vi "Sequencer Main - Copy.vi"() -> ()   [LabVIEW 2018] (continued)
                            }
                          }
                        }
                        frame 47 {
                          # "FALSE/Idle"
                          # "GoTo Test-nmb"
                          # "ReTest Cyckles"
                          # "RFID Case\nFTDI"
                          # "Test ADB LMS RFID"
                          n1783 = Unbundle By Name(w3499) -> ("Test Values.Upper Limit"=w3493:dbl, "Test Values.Lower Limit"=w3494:dbl, "Parameters"=w3496:string, "Step Description"=w3485:string)  [unwired: 1 out]
                          n1784 = property on="Tab Control Msg" class="TabCtl (strict)"("Value"=T4."Msg" ("Tab Control Msg")) -> (error out=w3497:errorcluster)  [unwired: 2 in, 1 out]
                          n1785 = in-place {
                            in-place-border: w3497 -> [_]
                            in-place-border: w3496 -> [w3545]
                            in-place-border: [w3539] -> w3495
                            in-place-border: w3494 -> [w3538]
                            in-place-border: w3493 -> [w3537]
                            in-place-border: [w3536] -> w3486
                            in-place-border: [w3534] -> w3492
                            in-place-border: w3485 -> [w3533]
                            in-place-border: [w3533] -> w3484
                            in-place-border: [w3532] -> w3483
                            n1786 = while {
                              shift-right: [w3613] -> _
                              shift-left: w3545 -> [w3614]
                              tunnel: [w3610] -> w3541 mode=indexing
                              stop <- w3612 stop-if-true
                              # "Get Array of Parametrs"
                              n1787 = Match Pattern(string=w3614, regular expression=">") -> (before substring=w3610:string, after substring=w3613:string, offset past match=w3611:i32)  [unwired: 1 in, 1 out]
                              n1788 = Less Than 0?(x=w3611) -> (x < 0?=w3612:bool)
                            }
                            n1789 = Index Array(array=w3541, index #1=0 ("index"), index #2=1 ("index"), index #3=2 ("index")) -> (element #1=w3535:string)  [unwired: 2 out]
                            n1790 = in-place {
                              in-place-border: [w3546] -> w3540
                              # "COMPORT OPEN?"
                              n1791 = global read "Global Variable.vi" "COM Port RFID"() -> (w3548:refnum<visa-resource-name>)
                              n1792 = Not Equal?(x=w3548, y="???") -> (x != y?=w3546:bool)
                            }
                            n1793 = while {
                              shift-right: [w3552] -> _
                              shift-left: w3535 -> [w3553]
                              tunnel: [w3549] -> w3534 mode=indexing
                              stop <- w3551 stop-if-true
                              # "Get Array of Sub Parametrs"
                              n1794 = Match Pattern(string=w3553, regular expression=":") -> (before substring=w3549:string, after substring=w3552:string, offset past match=w3550:i32)  [unwired: 1 in, 1 out]
                              n1795 = Less Or Equal To 0?(x=w3550) -> (x <= 0?=w3551:bool)
                            }
                            n1796 = case shown="True" w3540 {
                              tunnel: [FALSE w3569] -> w3539
                              tunnel: w3538 -> [_ w3571]
                              tunnel: w3537 -> [_ w3570]
                              tunnel: [w3555 w3560] -> w3536
                              tunnel: [w3555 w3559] -> w3532
                              frame False {
                                w3555 = "..."
                              }
                              frame True {
                                n1797 = flat-sequence {
                                tunnel: [w3590] -> w3563
                                tunnel: [w3591] -> w3562
                                tunnel: [w3589] -> w3561
                                tunnel: [w3589] -> w3558
                                tunnel: [w3609] -> w3565
                                tunnel: [w3600] -> w3567
                                tunnel: [w3599] -> w3566
                                tunnel: w3563 -> [w3605]
                                tunnel: w3562 -> [w3599]
                                tunnel: w3561 -> [w3598]
                                tunnel: [w3598] -> w3559
                                tunnel: w3558 -> [w3602]
                                tunnel: [w3596] -> w3557
                                frame #0 {
                                w3584 = "--------------------"
                                w3585 = "\r\n"
                                n1798 = case shown="True" FALSE {
                                frame False {
                                }
                                frame True {
                                n1799 = in-place {
                                # "Debug ONLY!"
                                n1800 = global write "Global Variable.vi" "Rd PID"("2205040012345") -> ()
                                }
                                }
                                }
                                n1801 = Concatenate Strings("Test ADB-LMS FRID M5", w3585, w3584, w3584, w3585) -> (w3586:string)
                                n1802 = property on="Msg Str" class="Str"("Value"=w3586) -> ()  [unwired: 2 in, 2 out]
                                }
                                frame #1 {
                                n1803 = global read "Global Variable.vi" "COM Port RFID"() -> (w3593:refnum<visa-resource-name>)
                                n1804 = call "pollingOnce.vi"("Rd Deelay"=u16 250 ("Delay"), "ComPort"=w3593) -> ("error out"=w3590:errorcluster, "rssi"=w3591:i16, "LMS"=w3589:string)  [unwired: 6 in, 1 out]
                                }
                                frame #2 {
                                w3594 = " (db) "
                                # "RFID PID"
                                n1805 = global read "Global Variable.vi" "Array Errors"() -> (w3608:errorcluster[])
                                n1806 = Number To Decimal String(number=w3599) -> (decimal integer string=w3595:string)  [unwired: 1 in]
                                n1807 = Match Pattern(string=w3602, regular expression="LED-LMS") -> (after substring=w3600:string)  [unwired: 1 in, 3 out]
                                n1808 = Replace Array Subset(array=w3608, new element=w3605, index=7) -> (w3607:errorcluster[])
                                n1809 = global write "Global Variable.vi" "Array Errors"(w3607) -> ()
                                n1810 = Concatenate Strings(w3595, w3594, "\r", "                   RFID-PID: " ("string"), w3600) -> (w3609:string)
                                n1811 = Concatenate Strings(w3598, " : ", w3595, w3594) -> (w3596:string)
                                }
                                }
                                n1812 = invoke on="Msg Str" class="Str" method="Append String"("string"=w3557) -> ()  [unwired: 3 in, 4 out]
                                n1813 = in-place {
                                in-place-border: [w3582] -> w3564
                                in-place-border: w3567 -> [w3581]
                                n1814 = global read "Global Variable.vi" "Baccode MEM"() -> (w3580:string)
                                n1815 = global write "Global Variable.vi" "Rd PID RFID"(w3581) -> ()
                                n1816 = Equal?(x=w3580, y=w3581) -> (x = y?=w3582:bool)
                                }
                                n1817 = case shown="False" w3564 {
                                tunnel: [w3574 w3575] -> w3560
                                tunnel: w3565 -> [w3573 w3575]
                                frame False {
                                n1818 = Concatenate Strings(w3573, " (False)" ("string")) -> (w3574:string)
                                }
                                frame True {
                                }
                                }
                                n1819 = in-place {
                                in-place-border: w3566 -> [w3577]
                                in-place-border: w3570 -> [w3579]
                                in-place-border: w3571 -> [w3578]
                                in-place-border: [w3576] -> w3568
                                n1820 = In Range and Coerce(upper limit=w3579, x=w3577, lower limit=w3578) -> (In Range?=w3576:bool)  [unwired: 1 out]
                                }
                                n1821 = And(x=w3568, y=w3564) -> (x .and. y?=w3569:bool)
                              }
                            }
                          }
                          n1822 = local read "Debugging"() -> (w3490:bool)
                          n1823 = in-place {
                            in-place-border: w3492 -> [w3525]
                            in-place-border: [w3524] -> w3491
                            in-place-border: [w3523] -> w3487
                            in-place-border: [w3522] -> w3488
                            # "Retest Parameters"
                            n1824 = Index Array(array=w3525, index #1=0 ("index"), index #2=1 ("index"), index #3=2 ("index")) -> (element #1=w3528:string, element #2=w3527:string, element #3=w3526:string)
                            n1825 = Decimal String To Number(string=w3526) -> (number=w3523:i32)  [unwired: 2 in, 1 out]
                            n1826 = Decimal String To Number(string=w3527) -> (number=w3522:i32)  [unwired: 2 in, 1 out]
                            n1827 = To Upper Case(1:w3528) -> (0:w3524:string)
                          }
                          n1828 = in-place {
                            in-place-border: [w3507] -> w3489
                            n1829 = global read "Global Variable.vi" "Retest Cnt"() -> (w3508:i16)
                            n1830 = Equal?(x=w3508, y=i16 0) -> (x = y?=w3507:bool)
                          }
                          n1831 = case shown="False" w3490 {
                            tunnel: w3491 -> [w3512 _]
                            tunnel: w3489 -> [w3509 _]
                            tunnel: w3487 -> [w3511 _]
                            tunnel: w3488 -> [w3510 _]
                            frame False {
                              # "Debug ?"
                              n1832 = case shown="\"FALSE\"" w3512 {
                                tunnel: w3509 -> [_ w3516]
                                tunnel: w3511 -> [_ w3513]
                                tunnel: w3510 -> [_ w3514]
                                frame "Idle", Default {
                                }
                                frame "FALSE" {
                                # "If \"false\" para exixst?"
                                n1833 = global write "Global Variable.vi" "Retest Step Nmb"(w3514) -> ()
                                n1834 = global write "Global Variable.vi" "Retest Nmb"(w3513) -> ()
                                n1835 = case shown="True" w3516 {
                                tunnel: w3513 -> [_ w3521]
                                frame False {
                                # "Else"
                                n1836 = global read "Global Variable.vi" "Retest Cnt"() -> (w3519:i16)
                                n1837 = Decrement(x=w3519) -> (x-1=w3518:i16)
                                n1838 = global write "Global Variable.vi" "Retest Cnt"(w3518) -> ()
                                n1839 = Wait (ms)(milliseconds to wait=u32 1000) -> ()  [unwired: 1 out]
                                }
                                frame True {
                                # "if(Retest-OFF & Cnt=0)"
                                n1840 = Decrement(x=w3521) -> (x-1=w3520:i32)
                                n1841 = global write "Global Variable.vi" "Retest Cnt"(w3520) -> ()
                                }
                                }
                                n1842 = global write "Global Variable.vi" "Retest ON"(TRUE ("Retest ON")) -> ()
                                }
                              }
                            }
                            frame True {
                            }
                          }
                          n1843 = in-place {
                            in-place-border: w3484 -> [w3503]
                            in-place-border: w3483 -> [w3502]
                            in-place-border: w3486 -> [w3501]
                            n1844 = call "Log Add Msg.vi"("Result"=w3501, "Communication"=w3502, "Description"=w3503) -> ("Out Msg"=w3504:string)
                            n1845 = property on="LogMsg" class="Str"("Text.Scroll Position"=inf) -> ()  [unwired: 2 in, 2 out]
                            n1846 = invoke on="LogMsg" class="Str" method="Append String"("string"=w3504) -> ()  [unwired: 3 in, 4 out]
                          }
                          n1847 = case shown="False" w3495 {
                            tunnel: [enum16{"Idle", "PASS", "FALSE"}."FALSE" ("Step Test Result") enum16{"Idle", "PASS", "FALSE"}."PASS" ("Step Test Result")] -> w3500
                            frame False {
                            }
                            frame True {
                            }
                          }
                        }
                        frame 50 {
                          # "Lover Lim"
                          # "Upper Lim"
                          # "PicoScope\n Case"
                          # "PicoScope Case"
                          n1848 = Unbundle By Name(w3634) -> ("Test Values.Upper Limit"=w3632:dbl, "Test Values.Lower Limit"=w3631:dbl, "Test Values.Numeric Value"=w3633:dbl)  [unwired: 1 out]
                          n1849 = property on="Tab Control Msg" class="TabCtl (strict)"("Value"=T21."Scope" ("Tab Control Msg")) -> (error out=w3630:errorcluster)  [unwired: 2 in, 1 out]
                          n1850 = flat-sequence {
                            tunnel: w3633 -> [w3667]
                            tunnel: w3632 -> [w3658]
                            tunnel: w3631 -> [w3657]
                            tunnel: w3630 -> [_]
                            tunnel: [w3658] -> w3621
                            tunnel: [w3657] -> w3620
                            tunnel: [w3676] -> w3629
                            tunnel: w3629 -> [w3695]
                            tunnel: [w3695] -> w3624
                            tunnel: [w3683] -> w3623
                            tunnel: [w3682] -> w3622
                            frame #0 {
                              n1851 = control-ref of="Channel B"() -> (w3660:refnum<vi>)
                              n1852 = control-ref of="Channel A"() -> (w3661:refnum<vi>)
                              n1853 = Multiply(x=w3657, y=-0.2) -> (x*y=w3662:dbl)
                              n1854 = Bundle("Lower Limit"=w3657, "Upper Limit"=w3658, "Numeric Value"=w3667) -> (w3668:T36)  [unwired: 1 in]
                              n1855 = Multiply(x=w3658, y=0.2) -> (x*y=w3664:dbl)
                              n1856 = Add(x=w3662, y=w3657) -> (x+y=w3659:dbl)
                              n1857 = property on="Limits" class="Slide (strict)"("Value"=w3668) -> ()  [unwired: 2 in, 2 out]
                              n1858 = invoke class="WFGraph (strict)" method="Reinit To Default"(reference=w3661) -> ()  [unwired: 2 in, 3 out]
                              n1859 = invoke class="WFGraph (strict)" method="Reinit To Default"(reference=w3660) -> ()  [unwired: 2 in, 3 out]
                              n1860 = Add(x=w3664, y=w3658) -> (x+y=w3663:dbl)
                              n1861 = property on="Limits" class="Slide (strict)"("Scale.Maximum"=w3663, "Scale.Minimum"=w3659) -> ()  [unwired: 2 in, 2 out]
                            }
                            frame #1 {
                              # "Ch B"
                              # "Ch A"
                              # "Trigger"
                              # "Err From PicoScope"
                              # "Read PicoScope"
                              n1862 = global read "Global Variable.vi" "Array Errors"() -> (w3675:errorcluster[])
                              n1863 = global read "Global Variable.vi" "PicoScope Max Adc Value"() -> (w3679:i16)
                              n1864 = global read "Global Variable.vi" "PicoScope Devi Info"() -> (w3680:T35)
                              n1865 = global read "Global Variable.vi" "PicoScope Handle"() -> (w3681:u32)
                              n1866 = Index Array(array=w3675, index=5) -> (element=w3674:errorcluster)
                              n1867 = control-ref of="Channel A"() -> (w3678:refnum<vi>)
                              n1868 = control-ref of="Channel B"() -> (w3677:refnum<vi>)
                              n1869 = call "PicoScope Read.vi"("WFD-Ref Ch-B"=w3677, "WFD-Ref Ch-A"=w3678, "Acquisition Settings"=T27 {"preTriggerSamples"=0, "postTriggerSamples"=1000, "timebase"=62500, "Down-Sample Mode"=0, "Down Sample Ratio"=1, "Oversample"=0}, "Trigger Settings"=T28 {"Trigger Enabled"=TRUE, "Trigger Source"=enum."Channel A", "Trigger Threshold (Volts)"=0.0, "Trigger Direction"=2, "Trigger Delay (samples)"=0, "Auto Trigger Time (ms)"=2000}, "Channel B Settings"=T26 {"Enabled"=TRUE, "Coupling"=0, "Range"=10, "Analogue Offset"=0.0}, "Channel A Settings"=T26 {"Enabled"=TRUE, "Coupling"=0, "Range"=10, "Analogue Offset"=0.0}, "error in"=w3674, "Max Adc value"=w3679, "Device Info"=w3680, "handle"=w3681) -> ("error out"=w3676:errorcluster)  [unwired: 1 in]
                            }
                            frame #2 {
                              w3684 = 11.25
                              # "Negative Vmin"
                              # "Positive Vmax"
                              # "Res Devider Compens\n100K / 10K"
                              # "Calculate Values"
                              n1870 = local read "Channel A"() -> (w3709:cluster{i32, dbl, dbl[]})
                              n1871 = local read "Channel B"() -> (w3702:cluster{i32, dbl, dbl[]})
                              n1872 = Unbundle(w3709) -> (w3706:dbl[])  [unwired: 2 out]
                              n1873 = Unbundle(w3702) -> (w3698:dbl[])  [unwired: 2 out]
                              n1874 = call-poly <vilib>:"Basic Averaged DC-RMS.vi"("signal in"=w3706) -> ("RMS value"=w3694:dbl, "DC value"=w3703:dbl)  [unwired: 7 in, 2 out]
                              n1875 = Array Max & Min(array=w3706) -> (max value=w3705:dbl, min value=w3704:dbl)  [unwired: 2 out]
                              n1876 = call-poly <vilib>:"Basic Averaged DC-RMS.vi"("signal in"=w3698) -> ("RMS value"=w3690:dbl, "DC value"=w3701:dbl)  [unwired: 7 in, 2 out]
                              n1877 = Array Max & Min(array=w3698) -> (max value=w3699:dbl, min value=w3700:dbl)  [unwired: 2 out]
                              n1878 = Subtract(x=w3705, y=w3703) -> (x-y=w3693:dbl)
                              n1879 = Add(x=w3704, y=w3703) -> (x+y=w3692:dbl)
                              n1880 = Subtract(x=w3699, y=w3701) -> (x-y=w3688:dbl)
                              n1881 = Add(x=w3700, y=w3701) -> (x+y=w3687:dbl)
                              n1882 = Multiply(x=w3694, y=w3684) -> (x*y=w3691:dbl)
                              n1883 = Multiply(x=w3693, y=w3684) -> (x*y=w3683:dbl)
                              n1884 = Multiply(x=w3692, y=w3684) -> (x*y=w3682:dbl)
                              n1885 = local read "Measure Ch-A"() -> (w3708:T10)
                              n1886 = Multiply(x=w3690, y=w3684) -> (x*y=w3689:dbl)
                              n1887 = Multiply(x=w3688, y=w3684) -> (x*y=w3686:dbl)
                              n1888 = Multiply(x=w3687, y=w3684) -> (x*y=w3685:dbl)
                              n1889 = local read "Measure Ch-B"() -> (w3696:T9)
                              n1890 = Bundle By Name(cluster=w3708, "MAX Vpp"=w3683, "PickToPoick / 2"=w3691, "MIN Vpp"=w3682) -> (w3707:T10)
                              n1891 = local write "Measure Ch-A"(w3707) -> ()
                              n1892 = Bundle By Name(cluster=w3696, "MAX Vpp"=w3686, "PickToPick / 2"=w3689, "MIN Vpp"=w3685) -> (w3697:T9)
                              n1893 = local write "Measure Ch-B"(w3697) -> ()
                            }
                          }
                          n1894 = global read "Global Variable.vi" "Array Errors"() -> (w3626:errorcluster[])
                          n1895 = Replace Array Subset(array=w3626, new element=w3624, index=5) -> (w3627:errorcluster[])
                          n1896 = in-place {
                            in-place-border: w3623 -> [w3638]
                            in-place-border: w3622 -> [w3637]
                            in-place-border: w3621 -> [w3647]
                            in-place-border: w3620 -> [w3646]
                            in-place-border: [w3648] -> w3619
                            in-place-border: [w3636] -> w3618
                            # "Step TEST Result"
                            n1897 = in-place {
                              in-place-border: w3647 -> [w3652]
                              in-place-border: w3646 -> [w3649]
                              in-place-border: [w3652] -> w3645
                              in-place-border: [w3651] -> w3643
                              in-place-border: [w3650] -> w3642
                              in-place-border: [w3649] -> w3644
                              n1898 = Multiply(x=w3649, y=-1.0) -> (x*y=w3650:dbl)
                              n1899 = Multiply(x=w3652, y=-1.0) -> (x*y=w3651:dbl)
                            }
                            n1900 = In Range and Coerce(upper limit=w3645, x=w3638, lower limit=w3644) -> (In Range?=w3641:bool)  [unwired: 1 out]
                            n1901 = In Range and Coerce(upper limit=w3642, x=w3637, lower limit=w3643) -> (In Range?=w3640:bool)  [unwired: 1 out]
                            n1902 = And(x=w3641, y=w3640) -> (x .and. y?=w3639:bool)
                            n1903 = Format Into String(format string="Max: %.1fVAC :: Min: %.1fVAC", w3638, w3637) -> (resulting string=w3636:string)  [unwired: 2 in, 1 out]
                            n1904 = case shown="False" w3639 {
                              tunnel: [enum16{"Idle", "PASS", "FALSE"}."FALSE" ("Step Test Result") enum16{"Idle", "PASS", "FALSE"}."PASS" ("Step Test Result")] -> w3648
                              frame False {
                              }
                              frame True {
                              }
                            }
                          }
                          n1905 = global write "Global Variable.vi" "Array Errors"(w3627) -> ()
                        }
                        frame 51 {
                          # "Create Thread Asynchronous"
                          # "PicoScope\n Case"
                          # "PicoScope Case"
                          n1906 = Unbundle By Name(w3726) -> ("Parameters"=w3713:string, "Test Values.Upper Limit"=w3724:dbl, "Test Values.Lower Limit"=w3723:dbl, "Test Values.Numeric Value"=w3725:dbl, "Step Description"=w3711:string)
                          n1907 = property on="Tab Control Msg" class="TabCtl (strict)"("Value"=T21."Msg" ("Tab Control Msg")) -> (error out=w3722:errorcluster)  [unwired: 2 in, 1 out]
                          n1908 = flat-sequence {
                            tunnel: w3725 -> [w3742]
                            tunnel: w3724 -> [w3733]
                            tunnel: w3723 -> [w3732]
                            tunnel: w3722 -> [_]
                            tunnel: [w3733] -> _
                            tunnel: [w3732] -> _
                            tunnel: w3713 -> [w3731]
                            tunnel: [w3730] -> w3712
                            tunnel: w3711 -> [w3729]
                            tunnel: [w3729] -> w3710
                            tunnel: [w3785] -> w3716
                            tunnel: w3712 -> [w3774]
                            tunnel: w3710 -> [w3759]
                            frame #0 {
                              n1909 = control-ref of="Channel B"() -> (w3735:refnum<vi>)
                              n1910 = control-ref of="Channel A"() -> (w3736:refnum<vi>)
                              n1911 = Multiply(x=w3732, y=-0.2) -> (x*y=w3737:dbl)
                              n1912 = Bundle("Lower Limit"=w3732, "Upper Limit"=w3733, "Numeric Value"=w3742) -> (w3743:T36)  [unwired: 1 in]
                              n1913 = while {
                                shift-right: [w3747] -> _
                                shift-left: w3731 -> [w3748]
                                tunnel: [w3744] -> w3730 mode=indexing
                                stop <- w3746 stop-if-true
                                # "Get Array of Parametrs"
                                n1914 = Match Pattern(string=w3748, regular expression=">") -> (before substring=w3744:string, after substring=w3747:string, offset past match=w3745:i32)  [unwired: 1 in, 1 out]
                                n1915 = Less Than 0?(x=w3745) -> (x < 0?=w3746:bool)
                              }
                              n1916 = Multiply(x=w3733, y=0.2) -> (x*y=w3739:dbl)
                              n1917 = Add(x=w3737, y=w3732) -> (x+y=w3734:dbl)
                              n1918 = property on="Limits" class="Slide (strict)"("Value"=w3743) -> ()  [unwired: 2 in, 2 out]
                              n1919 = Add(x=w3739, y=w3733) -> (x+y=w3738:dbl)
                              n1920 = invoke class="WFGraph (strict)" method="Reinit To Default"(reference=w3736) -> ()  [unwired: 2 in, 3 out]
                              n1921 = invoke class="WFGraph (strict)" method="Reinit To Default"(reference=w3735) -> ()  [unwired: 2 in, 3 out]
                              n1922 = property on="Limits" class="Slide (strict)"("Scale.Maximum"=w3738, "Scale.Minimum"=w3734) -> ()  [unwired: 2 in, 2 out]
                            }
                            frame #1 {
                              w3757 = "----------------------"
                              w3758 = "\r\n"
                              # "Ch B"
                              # "Ch A"
                              # "Trigger"
                              # "Read PicoScope"
                              n1923 = Index Array(array=w3774, index #1=0 ("index"), index #2=1 ("index"), index #3=2 ("index")) -> (element #1=w3770:string, element #2=w3764:string, element #3=w3762:string)
                              n1924 = vi-ref "PicoScope Read.vi"() -> (w3754:refnum<vi>)
                              n1925 = property class="VI"(reference=w3754) -> (error out=w3751:errorcluster, "Path"=w3753:path)  [unwired: 1 in, 1 out]
                              n1926 = Decimal String To Number(string=w3764) -> (number=w3767:i32)  [unwired: 2 in, 1 out]
                              n1927 = Decimal String To Number(string=w3762) -> (number=w3766:i32)  [unwired: 2 in, 1 out]
                              n1928 = global read "Global Variable.vi" "PicoScope Max Adc Value"() -> (w3779:i16)
                              n1929 = case shown="\"A\", Default" w3770 {
                                tunnel: [T28 {"Trigger Enabled"=TRUE, "Trigger Source"=enum."Channel A", "Trigger Threshold (Volts)"=0.1, "Trigger Direction"=2, "Trigger Delay (samples)"=0, "Auto Trigger Time (ms)"=2000} ("Trigger Settings") T28 {"Trigger Enabled"=TRUE, "Trigger Source"=enum."Channel B", "Trigger Threshold (Volts)"=0.1, "Trigger Direction"=2, "Trigger Delay (samples)"=0, "Auto Trigger Time (ms)"=3000} ("Trigger Settings")] -> w3756
                                tunnel: ["Trig: Ch-A" "Trig: Ch-B"] -> w3760
                                frame "A", Default {
                                }
                                frame "B" {
                                }
                              }
                              n1930 = global read "Global Variable.vi" "PicoScope Devi Info"() -> (w3780:T35)
                              n1931 = global read "Global Variable.vi" "PicoScope Handle"() -> (w3781:u32)
                              n1932 = Open VI Reference(type specifier VI Refnum (for type only)=refnum<vi> refnum, vi path=w3753, options=128, error in (no error)=w3751) -> (vi reference=w3784:refnum<vi>, error out=w3783:errorcluster)  [unwired: 2 in]
                              n1933 = Bundle By Name(cluster=T27 {"preTriggerSamples"=500, "postTriggerSamples"=8000, "timebase"=1000, "Down-Sample Mode"=0, "Down Sample Ratio"=1, "Oversample"=0} ("Acquisition Settings"), "postTriggerSamples"=w3767, "timebase"=w3766) -> (w3768:T27)
                              n1934 = control-ref of="Channel A"() -> (w3775:refnum<vi>)
                              n1935 = control-ref of="Channel B"() -> (w3777:refnum<vi>)
                              n1936 = call-by-ref "Start Asynchronous Call"(reference=w3784, error in=w3783, "WFD-Ref Ch-B"=w3777, "WFD-Ref Ch-A"=w3775, "Acquisition Settings"=w3768, "Trigger Settings"=w3756, "Channel B Settings"=T26 {"Enabled"=TRUE, "Coupling"=0, "Range"=6, "Analogue Offset"=0.0}, "Channel A Settings"=T26 {"Enabled"=TRUE, "Coupling"=0, "Range"=6, "Analogue Offset"=0.0}, "Max Adc value"=w3779, "Device Info"=w3780, "handle"=w3781) -> (reference out=w3776:refnum<vi>, error out=w3750:errorcluster)  [unwired: 2 in, 1 out]
                              n1937 = case shown="Error" w3750 {
                                frame No Error {
                                }
                                frame Error {
                                n1938 = One Button Dialog(message="PycoScope Err") -> ()  [unwired: 1 in, 1 out]
                                }
                              }
                              n1939 = Concatenate Strings(w3759, w3758, w3757, w3757, w3758, w3760, w3758, "Samples: ", w3764, w3758, "Base Time: ", w3762, w3758) -> (w3761:string)
                              n1940 = Close Reference(reference=w3776, error in (no error)=w3750) -> (error out=w3785:errorcluster)
                              n1941 = local write "Msg Str"(w3761) -> ()
                            }
                          }
                          n1942 = global read "Global Variable.vi" "Array Errors"() -> (w3719:errorcluster[])
                          n1943 = Replace Array Subset(array=w3719, new element=w3716, index=5) -> (w3720:errorcluster[])
                          n1944 = global write "Global Variable.vi" "Array Errors"(w3720) -> ()
                          n1945 = Unbundle By Name(w3716) -> ("status"=w3715:bool)
                          n1946 = Not(x=w3715) -> (.not. x?=w3714:bool)
                          n1947 = case shown="True" w3714 {
                            tunnel: [enum16{"Idle", "PASS", "FALSE"}."FALSE" ("Step Test Result") enum16{"Idle", "PASS", "FALSE"}."Idle" ("Step Test Result")] -> w3717
                            frame False {
                            }
                            frame True {
                            }
                          }
                        }
                        frame 52 {
                          # "Read Positive & negative Values"
                          # "Lover Lim"
                          # "Upper Lim"
                          # "PicoScope\n Case"
                          # "PicoScope Case"
                          n1948 = Unbundle By Name(w3813) -> ("Parameters"=w3807:string, "Test Values.Upper Limit"=w3811:dbl, "Test Values.Lower Limit"=w3810:dbl, "Test Values.Numeric Value"=w3812:dbl)
                          n1949 = property on="Tab Control Msg" class="TabCtl (strict)"("Value"=T21."Scope" ("Tab Control Msg")) -> (error out=w3809:errorcluster)  [unwired: 2 in, 1 out]
                          n1950 = flat-sequence {
                            tunnel: w3812 -> [w3851]
                            tunnel: w3811 -> [w3844]
                            tunnel: w3810 -> [w3843]
                            tunnel: w3809 -> [_]
                            tunnel: [w3844] -> w3797
                            tunnel: [w3843] -> w3798
                            tunnel: w3807 -> [w3842]
                            tunnel: [w3840] -> w3802
                            tunnel: [w3836] -> w3799
                            tunnel: [w3904] -> w3806
                            tunnel: [w3903] -> w3805
                            tunnel: [w3902] -> w3804
                            tunnel: [w3901] -> w3803
                            tunnel: w3802 -> [w3893]
                            tunnel: [w3893] -> w3801
                            tunnel: [w3892] -> w3800
                            tunnel: w3799 -> [w3892]
                            tunnel: w3806 -> [w3924]
                            tunnel: w3805 -> [w3923]
                            tunnel: w3804 -> [w3922]
                            tunnel: w3803 -> [w3921]
                            tunnel: w3801 -> [w3939]
                            tunnel: w3800 -> [w3932]
                            tunnel: [w3916] -> w3795
                            tunnel: [w3915] -> w3793
                            tunnel: [w3957] -> w3796
                            tunnel: w3795 -> [w3957]
                            tunnel: [w3956] -> w3794
                            tunnel: w3793 -> [w3956]
                            frame #0 {
                              n1951 = while {
                                shift-right: [w3862] -> _
                                shift-left: w3842 -> [w3863]
                                tunnel: [w3859] -> w3841 mode=indexing
                                stop <- w3861 stop-if-true
                                # "Get Array of Parametrs"
                                n1952 = Match Pattern(string=w3863, regular expression=">") -> (before substring=w3859:string, after substring=w3862:string, offset past match=w3860:i32)  [unwired: 1 in, 1 out]
                                n1953 = Less Than 0?(x=w3860) -> (x < 0?=w3861:bool)
                              }
                              n1954 = Multiply(x=w3843, y=-0.2) -> (x*y=w3846:dbl)
                              n1955 = Bundle("Lower Limit"=w3843, "Upper Limit"=w3844, "Numeric Value"=w3851) -> (w3852:T36)  [unwired: 1 in]
                              n1956 = Multiply(x=w3844, y=0.2) -> (x*y=w3848:dbl)
                              n1957 = Add(x=w3846, y=w3843) -> (x+y=w3845:dbl)
                              n1958 = property on="Limits" class="Slide (strict)"("Value"=w3852) -> ()  [unwired: 2 in, 2 out]
                              n1959 = Add(x=w3848, y=w3844) -> (x+y=w3847:dbl)
                              n1960 = property on="Limits" class="Slide (strict)"("Scale.Maximum"=w3847, "Scale.Minimum"=w3845) -> ()  [unwired: 2 in, 2 out]
                              n1961 = Index Array(array=w3841, index #1=0 ("index"), index #2=1 ("index")) -> (element #1=w3840:string, element #2=w3837:string)
                              n1962 = while {
                                shift-right: [w3856] -> _
                                shift-left: w3837 -> [w3857]
                                tunnel: [w3853] -> w3836 mode=indexing
                                stop <- w3855 stop-if-true
                                # "Get Array of Sub Parametrs"
                                n1963 = Match Pattern(string=w3857, regular expression=":") -> (before substring=w3853:string, after substring=w3856:string, offset past match=w3854:i32)  [unwired: 1 in, 1 out]
                                n1964 = Less Than 0?(x=w3854) -> (x < 0?=w3855:bool)
                              }
                            }
                            frame #1 {
                              w3865 = TRUE
                              w3896 = 100 ("index")
                              # "700"
                              # "302"
                              # "Devider compensite"
                              # "remove first\nxx element (noise)"
                              # "Ch-B Negative Vmin"
                              # "Ch-B Positive Vmax"
                              # "Ch-A Negative Vmin"
                              # "Ch-A Positive Vmax"
                              # "Res Devider Compens\n100K / 10K"
                              # "Calculate Values"
                              n1965 = local read "Channel A"() -> (w3889:cluster{i32, dbl, dbl[]})
                              n1966 = local read "Channel B"() -> (w3886:cluster{i32, dbl, dbl[]})
                              n1967 = Unbundle(w3889) -> (w3894:dbl[])  [unwired: 2 out]
                              n1968 = Unbundle(w3886) -> (w3898:dbl[])  [unwired: 2 out]
                              n1969 = Array Size(array=w3894) -> (size(s)=w3900:i32)
                              n1970 = Array Size(array=w3898) -> (size(s)=w3897:i32)
                              n1971 = Subtract(x=w3900, y=w3896) -> (x-y=w3899:i32)
                              n1972 = Array Subset(array=w3894, index=w3896, length=w3899) -> (w3877:dbl[])
                              n1973 = Add(x=290, y="Correction") -> (x+y=w3878:i32)
                              "Pico Scope Correction" <- w3878
                              n1974 = Subtract(x=w3897, y=w3896) -> (x-y=w3895:i32)
                              n1975 = Array Subset(array=w3898, index=w3896, length=w3895) -> (w3891:dbl[])
                              n1976 = call "Wave Filter.vi"("Filter ON"=w3865, "Value"="F-Value", "Data In"=w3877) -> ("Data Out"=w3887:dbl[])  [unwired: 8 in]
                              n1977 = call "Wave Filter.vi"("Filter ON"=w3865, "Value"="F-Value", "Data In"=w3891) -> ("Data Out"=w3882:dbl[])  [unwired: 8 in]
                              n1978 = call "Convert to Dynamic Data"("Array"=w3887) -> ("Dynamic Data Type"=w3874:dynamicdata)  [unwired: 3 in]
                              n1979 = call "Convert to Dynamic Data2"("Array"=w3882) -> ("Dynamic Data Type"=w3873:dynamicdata)  [unwired: 3 in]
                              n1980 = Bundle(cluster=w3886, w3882) -> (w3885:cluster{i32, dbl, dbl[]})  [unwired: 2 in]
                              n1981 = call "Amplitude and Level Measurements2"("Signals"=w3873) -> ("Mean (DC)"=w3875:dynamicdata, "Negative Peak"=w3880:dynamicdata, "Positive Peak"=w3881:dynamicdata, "Peak to Peak"=w3871:dynamicdata)  [unwired: 10 in, 1 out]
                              n1982 = Bundle(cluster=w3889, w3887) -> (w3888:cluster{i32, dbl, dbl[]})  [unwired: 2 in]
                              n1983 = call "Amplitude and Level Measurements"("Signals"=w3874) -> ("Mean (DC)"=w3876:dynamicdata, "Negative Peak"=w3883:dynamicdata, "Positive Peak"=w3884:dynamicdata, "Peak to Peak"=w3868:dynamicdata)  [unwired: 10 in, 1 out]
                              n1984 = local write "Channel B"(w3885) -> ()
                              n1985 = Divide(x=w3868, y=2.0) -> (x/y=w3867:dynamicdata)
                              n1986 = Divide(x=w3871, y=2.0) -> (x/y=w3870:dynamicdata)
                              n1987 = local write "Channel A"(w3888) -> ()
                              n1988 = Subtract(1:w3876, 2:w3884) -> (0:w3910:dynamicdata)  [unwired: 1 in, 1 out]
                              n1989 = Add(1:w3876, 2:w3883) -> (0:w3909:dynamicdata)  [unwired: 1 in, 1 out]
                              n1990 = Subtract(1:w3875, 2:w3881) -> (0:w3906:dynamicdata)  [unwired: 1 in, 1 out]
                              n1991 = Add(1:w3875, 2:w3880) -> (0:w3905:dynamicdata)  [unwired: 1 in, 1 out]
                              n1992 = Multiply(x=w3867, y=w3878) -> (x*y=w3908:dynamicdata)
                              n1993 = Multiply(x=w3910, y=w3878) -> (x*y=w3904:dynamicdata)
                              n1994 = Multiply(x=w3909, y=w3878) -> (x*y=w3903:dynamicdata)
                              n1995 = local read "Measure Ch-A"() -> (w3914:T10)
                              n1996 = Multiply(x=w3870, y=w3878) -> (x*y=w3907:dynamicdata)
                              n1997 = Multiply(x=w3906, y=w3878) -> (x*y=w3902:dynamicdata)
                              n1998 = Multiply(x=w3905, y=w3878) -> (x*y=w3901:dynamicdata)
                              n1999 = Bundle By Name(cluster=w3914, "MAX Vpp"=w3904, "PickToPoick / 2"=w3908, "MIN Vpp"=w3903) -> (w3913:T10)
                              n2000 = local read "Measure Ch-B"() -> (w3911:T9)
                              n2001 = Bundle By Name(cluster=w3911, "MAX Vpp"=w3902, "PickToPick / 2"=w3907, "MIN Vpp"=w3901) -> (w3912:T9)
                              n2002 = local write "Measure Ch-B"(w3912) -> ()
                              n2003 = local write "Measure Ch-A"(w3913) -> ()
                            }
                            frame #2 {
                              # "GoTo Test-nmb"
                              # "ReTest Cyckles"
                              # "Select Channel & Set Retest Parametrs in FALSE Case"
                              n2004 = Index Array(array=w3932, index #1=0 ("index"), index #2=1 ("index"), index #3=2 ("index")) -> (element #1=w3936:string, element #2=w3937:string, element #3=w3938:string)
                              n2005 = global read "Global Variable.vi" "Retest Cnt"() -> (w3931:i16)
                              n2006 = local read "Debugging"() -> (w3929:bool)
                              n2007 = To Upper Case(1:w3936) -> (0:w3928:string)
                              n2008 = call "Convert from Dynamic Data"("Dynamic Data Type"=w3924) -> ("Scalar"=w3920:dbl)  [unwired: 3 in]
                              n2009 = call "Convert from Dynamic Data2"("Dynamic Data Type"=w3923) -> ("Scalar"=w3919:dbl)  [unwired: 3 in]
                              n2010 = call "Convert from Dynamic Data3"("Dynamic Data Type"=w3922) -> ("Scalar"=w3918:dbl)  [unwired: 3 in]
                              n2011 = call "Convert from Dynamic Data4"("Dynamic Data Type"=w3921) -> ("Scalar"=w3917:dbl)  [unwired: 3 in]
                              n2012 = Decimal String To Number(string=w3938) -> (number=w3925:i32)  [unwired: 2 in, 1 out]
                              n2013 = Decimal String To Number(string=w3937) -> (number=w3927:i32)  [unwired: 2 in, 1 out]
                              n2014 = Equal?(x=w3931, y=i16 0) -> (x = y?=w3926:bool)
                              n2015 = case shown="False" w3929 {
                                tunnel: w3928 -> [w3943 _]
                                tunnel: w3926 -> [w3940 _]
                                tunnel: w3925 -> [w3942 _]
                                tunnel: w3927 -> [w3941 _]
                                frame False {
                                n2016 = case shown="\"FALSE\"" w3943 {
                                tunnel: w3940 -> [_ w3947]
                                tunnel: w3942 -> [_ w3944]
                                tunnel: w3941 -> [_ w3945]
                                frame "Idle", Default {
                                }
                                frame "FALSE" {
                                n2017 = global write "Global Variable.vi" "Retest Step Nmb"(w3945) -> ()
                                n2018 = global write "Global Variable.vi" "Retest Nmb"(w3944) -> ()
                                n2019 = case shown="True" w3947 {
                                tunnel: w3944 -> [_ w3951]
                                tunnel: w3945 -> [_ _]
                                frame False {
                                n2020 = global read "Global Variable.vi" "Retest Cnt"() -> (w3949:i16)
                                n2021 = Decrement(x=w3949) -> (x-1=w3948:i16)
                                n2022 = global write "Global Variable.vi" "Retest Cnt"(w3948) -> ()
                                }
                                frame True {
                                # "if(Retest-OFF & Cnt=0)"
                                n2023 = Decrement(x=w3951) -> (x-1=w3950:i32)
                                n2024 = global write "Global Variable.vi" "Retest Cnt"(w3950) -> ()
                                }
                                }
                                n2025 = global write "Global Variable.vi" "Retest ON"(TRUE ("Retest ON")) -> ()
                                }
                                }
                                }
                                frame True {
                                }
                              }
                              n2026 = case shown="\"A\", Default" w3939 {
                                tunnel: [w3953 w3955] -> w3916
                                tunnel: w3920 -> [w3953 _]
                                tunnel: w3919 -> [w3952 _]
                                tunnel: [w3952 w3954] -> w3915
                                tunnel: w3918 -> [_ w3955]
                                tunnel: w3917 -> [_ w3954]
                                frame "A", Default {
                                }
                                frame "B" {
                                }
                              }
                            }
                            frame #3 {
                              # "Negative MIN"
                              # "Positive MAX"
                              n2027 = Multiply(x="Delay", y=u32 1000 ("milliseconds to wait")) -> (x*y=w3958:u32)
                              n2028 = Wait (ms)(milliseconds to wait=w3958) -> ()  [unwired: 1 out]
                            }
                          }
                          n2029 = in-place {
                            in-place-border: w3796 -> [w3820]
                            in-place-border: w3794 -> [w3819]
                            in-place-border: w3797 -> [w3826]
                            in-place-border: w3798 -> [w3825]
                            in-place-border: [w3827] -> w3792
                            in-place-border: [w3818] -> w3791
                            # "Step Result Msg"
                            # "Step TEST Result"
                            n2030 = in-place {
                              in-place-border: w3826 -> [w3831]
                              in-place-border: w3825 -> [w3828]
                              in-place-border: [w3831] -> w3824
                              in-place-border: [w3830] -> w3822
                              in-place-border: [w3829] -> w3821
                              in-place-border: [w3828] -> w3823
                              n2031 = Multiply(x=w3828, y=-1.0) -> (x*y=w3829:dbl)
                              n2032 = Multiply(x=w3831, y=-1.0) -> (x*y=w3830:dbl)
                            }
                            n2033 = In Range and Coerce(upper limit=w3824, x=w3820, lower limit=w3823) -> (In Range?=w3816:bool)  [unwired: 1 out]
                            n2034 = In Range and Coerce(upper limit=w3821, x=w3819, lower limit=w3822) -> (In Range?=w3815:bool)  [unwired: 1 out]
                            n2035 = And(x=w3816, y=w3815) -> (x .and. y?=w3814:bool)
                            n2036 = case shown="False" w3814 {
                              tunnel: [enum16{"Idle", "PASS", "FALSE"}."FALSE" ("Step Test Result") enum16{"Idle", "PASS", "FALSE"}."PASS" ("Step Test Result")] -> w3827
                              frame False {
                              }
                              frame True {
                              }
                            }
                            n2037 = Format Into String(format string="Max: %.1fVAC :: Min: %.1fVAC", w3820, w3819) -> (resulting string=w3818:string)  [unwired: 2 in, 1 out]
                          }
                        }
                        frame 56 {
                          # "Read Peack To Peak / 2"
                          # "Lover Lim"
                          # "Upper Lim"
                          # "PicoScope"
                          # "PicoScope Case"
                          n2038 = Unbundle By Name(w3979) -> ("Parameters"=w3973:string, "Test Values.Upper Limit"=w3977:dbl, "Test Values.Lower Limit"=w3976:dbl, "Test Values.Numeric Value"=w3978:dbl)
                          n2039 = property on="Tab Control Msg" class="TabCtl (strict)"("Value"=T21."Scope" ("Tab Control Msg")) -> (error out=w3975:errorcluster)  [unwired: 2 in, 1 out]
                          n2040 = flat-sequence {
                            tunnel: w3978 -> [w4006]
                            tunnel: w3977 -> [w3999]
                            tunnel: w3976 -> [w3998]
                            tunnel: w3975 -> [_]
                            tunnel: [w3999] -> w3965
                            tunnel: [w3998] -> w3966
                            tunnel: w3973 -> [w3997]
                            tunnel: [w3995] -> w3970
                            tunnel: [w3991] -> w3967
                            tunnel: [w4025] -> w3972
                            tunnel: [w4024] -> w3971
                            tunnel: w3970 -> [w4050]
                            tunnel: [w4050] -> w3969
                            tunnel: [w4049] -> w3968
                            tunnel: w3967 -> [w4049]
                            tunnel: w3972 -> [w4074]
                            tunnel: w3971 -> [w4073]
                            tunnel: w3969 -> [w4089]
                            tunnel: w3968 -> [w4082]
                            tunnel: [w4072] -> w3963
                            tunnel: [w4105] -> w3964
                            tunnel: w3963 -> [w4105]
                            frame #0 {
                              n2041 = while {
                                shift-right: [w4017] -> _
                                shift-left: w3997 -> [w4018]
                                tunnel: [w4014] -> w3996 mode=indexing
                                stop <- w4016 stop-if-true
                                # "Get Array of Parametrs"
                                n2042 = Match Pattern(string=w4018, regular expression=">") -> (before substring=w4014:string, after substring=w4017:string, offset past match=w4015:i32)  [unwired: 1 in, 1 out]
                                n2043 = Less Than 0?(x=w4015) -> (x < 0?=w4016:bool)
                              }
                              n2044 = Multiply(x=w3998, y=-0.2) -> (x*y=w4001:dbl)
                              n2045 = Bundle("Lower Limit"=w3998, "Upper Limit"=w3999, "Numeric Value"=w4006) -> (w4007:T36)  [unwired: 1 in]
                              n2046 = Multiply(x=w3999, y=0.2) -> (x*y=w4003:dbl)
                              n2047 = Add(x=w4001, y=w3998) -> (x+y=w4000:dbl)
                              n2048 = property on="Limits" class="Slide (strict)"("Value"=w4007) -> ()  [unwired: 2 in, 2 out]
                              n2049 = Add(x=w4003, y=w3999) -> (x+y=w4002:dbl)
                              n2050 = property on="Limits" class="Slide (strict)"("Scale.Maximum"=w4002, "Scale.Minimum"=w4000) -> ()  [unwired: 2 in, 2 out]
                              n2051 = Index Array(array=w3996, index #1=0 ("index"), index #2=1 ("index")) -> (element #1=w3995:string, element #2=w3992:string)
                              n2052 = while {
                                shift-right: [w4011] -> _
                                shift-left: w3992 -> [w4012]
                                tunnel: [w4008] -> w3991 mode=indexing
                                stop <- w4010 stop-if-true
                                # "Get Array of Sub Parametrs"
                                n2053 = Match Pattern(string=w4012, regular expression=":") -> (before substring=w4008:string, after substring=w4011:string, offset past match=w4009:i32)  [unwired: 1 in, 1 out]
                                n2054 = Less Than 0?(x=w4009) -> (x < 0?=w4010:bool)
                              }
                            }
                            frame #1 {
                              w4020 = TRUE
                              w4053 = 100 ("index")
                              # "700"
                              # "Devider compensite"
                              # "remove first\nxx element (noise)"
                              # "Ch-B Peack To Peack / 2"
                              # "Ch-A Peack To Peack / 2"
                              # "Res Devider Compens\n100K / 10K"
                              # "Calculate Values"
                              n2055 = local read "Correction"() -> (w4023:i32)
                              n2056 = local read "Channel A"() -> (w4047:cluster{i32, dbl, dbl[]})
                              n2057 = local read "Channel B"() -> (w4044:cluster{i32, dbl, dbl[]})
                              n2058 = Unbundle(w4047) -> (w4051:dbl[])  [unwired: 2 out]
                              n2059 = Unbundle(w4044) -> (w4055:dbl[])  [unwired: 2 out]
                              n2060 = local read "F-Value"() -> (w4021:dbl)
                              n2061 = Array Size(array=w4051) -> (size(s)=w4057:i32)
                              n2062 = Array Size(array=w4055) -> (size(s)=w4054:i32)
                              n2063 = Subtract(x=w4057, y=w4053) -> (x-y=w4056:i32)
                              n2064 = Array Subset(array=w4051, index=w4053, length=w4056) -> (w4036:dbl[])
                              n2065 = Add(x=290, y=w4023) -> (x+y=w4022:i32)
                              n2066 = Subtract(x=w4054, y=w4053) -> (x-y=w4052:i32)
                              n2067 = Array Subset(array=w4055, index=w4053, length=w4052) -> (w4048:dbl[])
                              n2068 = call "Wave Filter.vi"("Filter ON"=w4020, "Value"=w4021, "Data In"=w4036) -> ("Data Out"=w4045:dbl[])  [unwired: 8 in]
                              n2069 = call "Wave Filter.vi"("Filter ON"=w4020, "Value"=w4021, "Data In"=w4048) -> ("Data Out"=w4040:dbl[])  [unwired: 8 in]
                              n2070 = local write "Pico Scope Correction"(w4022) -> ()
                              n2071 = call "Convert to Dynamic Data4"("Array"=w4045) -> ("Dynamic Data Type"=w4033:dynamicdata)  [unwired: 3 in]
                              n2072 = call "Convert to Dynamic Data3"("Array"=w4040) -> ("Dynamic Data Type"=w4032:dynamicdata)  [unwired: 3 in]
                              n2073 = Bundle(cluster=w4044, w4040) -> (w4043:cluster{i32, dbl, dbl[]})  [unwired: 2 in]
                              n2074 = call "Amplitude and Level Measurements4"("Signals"=w4032) -> ("Mean (DC)"=w4034:dynamicdata, "Negative Peak"=w4038:dynamicdata, "Positive Peak"=w4039:dynamicdata, "Peak to Peak"=w4031:dynamicdata)  [unwired: 10 in, 1 out]
                              n2075 = Bundle(cluster=w4047, w4045) -> (w4046:cluster{i32, dbl, dbl[]})  [unwired: 2 in]
                              n2076 = call "Amplitude and Level Measurements3"("Signals"=w4033) -> ("Mean (DC)"=w4035:dynamicdata, "Negative Peak"=w4041:dynamicdata, "Positive Peak"=w4042:dynamicdata, "Peak to Peak"=w4028:dynamicdata)  [unwired: 10 in, 1 out]
                              n2077 = local write "Channel B"(w4043) -> ()
                              n2078 = Divide(x=w4028, y=2.0) -> (x/y=w4027:dynamicdata)
                              n2079 = Divide(x=w4031, y=2.0) -> (x/y=w4030:dynamicdata)
                              n2080 = local write "Channel A"(w4046) -> ()
                              n2081 = Subtract(1:w4035, 2:w4042) -> (0:w4065:dynamicdata)  [unwired: 1 in, 1 out]
                              n2082 = Add(1:w4035, 2:w4041) -> (0:w4064:dynamicdata)  [unwired: 1 in, 1 out]
                              n2083 = Subtract(1:w4034, 2:w4039) -> (0:w4063:dynamicdata)  [unwired: 1 in, 1 out]
